vi "liftCellOrPullPatch-v02.vi"(0 "which manipulator":T5(ring), 1 "controls array in":refnum<vi>[](array[refnum]), 5 "LiftCell?":bool, 7 "set pressure (mBar)":dbl format="%#_13g", 11 "error in":errorcluster, 12 "common cluster":T4, 13 "individual controls in":T3, 14 "images":T1) -> (3 "control array out":refnum<vi>[](array[refnum]), 15 "error out":errorcluster)   [LabVIEW 2019]
uses:
  multipatch/controls/multipatch_common_controls_v4.ctl
  machine_vision/controls/transform_cluster_actuator.ctl
  machine_vision/coordinate model vis/transform_properties_actuators.ctl
  pipette cleaning/pressure box/cleaning_soft/controls/actuator_cluster.ctl
  pipette cleaning/pressure box/cleaning_soft/controls/actuator_type.ctl
  pipette cleaning/pressure box/cleaning_soft/controls/pressure_box_control.ctl
  pipette cleaning/pressure box/cleaning_soft/controls/pressure_box_type.ctl
  controls/NH_method.ctl
  multipatch/controls/multipatch_individual_controls_v5.ctl
  controls/memtest_def.ctl
  multipatch/controls/images_controls.ctl
  <vilib>/vision/Image Controls.llb/IMAQ Image.ctl
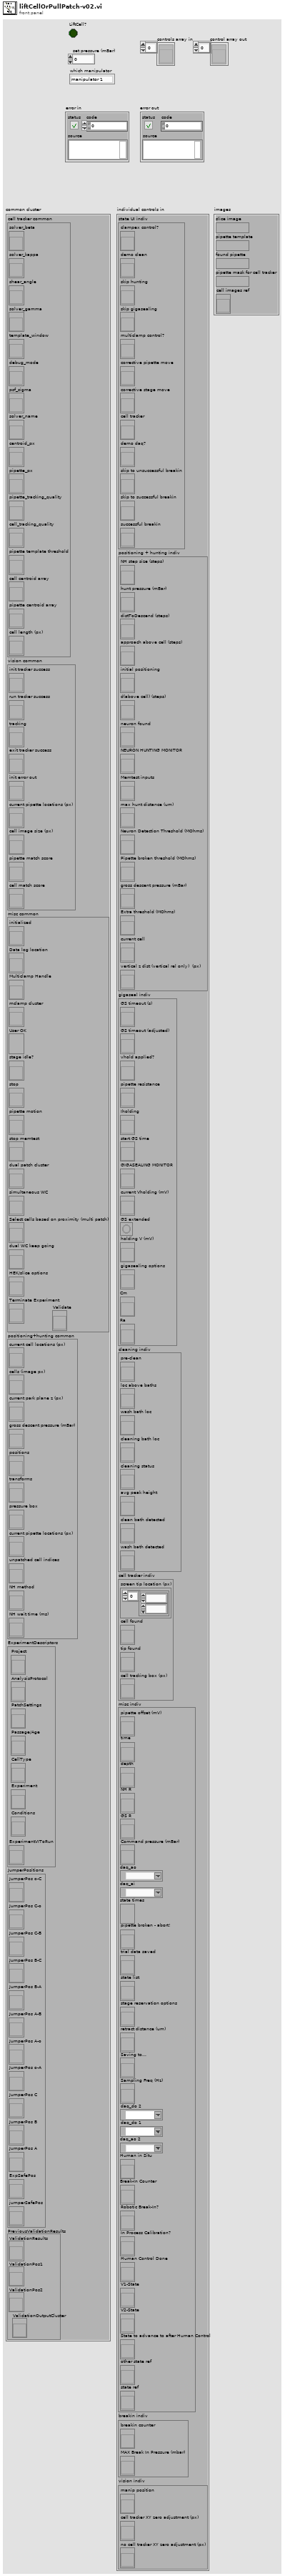
[diagram p1: front panel]
types:
  T1 = typedef "images_controls.ctl" = cluster{"slice image":T2, "pipette template":T2, "found pipette":T2, "pipette mask for cell tracker":T2, "cell images ref":refnum<vi>}
  T2 = typedef "IMAQ Image.ctl" = refnum<image>
  T3 = typedef "multipatch_individual_controls_v5.ctl" = cluster{"state UI indiv":cluster{"clampex control?":refnum<vi>, "demo clean":refnum<vi>, "skip hunting":refnum<vi>, "skip gigasealing":refnum<vi>, "multiclamp control?":refnum<vi>, "corrective pipette move":refnum<vi>, "corrective stage move":refnum<vi>, "cell tracker":refnum<vi>, "demo daq?":refnum<vi>, "skip to unsuccessful breakin":refnum<vi>, "skip to successful breakin":refnum<vi>, "successful breakin":refnum<vi>}, "positioning + hunting indiv":cluster{"NH step size (steps)":refnum<vi>, "hunt pressure (mBar)":refnum<vi>, "distToDescend (steps)":refnum<vi>, "approach above cell (steps)":refnum<vi>, "initial positioning":refnum<vi>, "d(above cell) (steps)":refnum<vi>, "neuron found":refnum<vi>, "NEURON HUNTING MONITOR":refnum<vi>, "Memtest inputs":refnum<vi>, "max hunt distance (um)":refnum<vi>, "Neuron Detection Threshold (MOhms)":refnum<vi>, "Pipette broken threshold (MOhms)":refnum<vi>, "gross descent pressure (mBar)":refnum<vi>, "Extra threshold (MOhms)":refnum<vi>, "current cell":refnum<vi>, "vertical z dist (vertical rel only)  (px)":refnum<vi>}, "gigaseal indiv":cluster{"GS timeout (s)":refnum<vi>, "GS timeout (adjusted)":refnum<vi>, "vhold applied?":refnum<vi>, "pipette resistance":refnum<vi>, "Iholding":refnum<vi>, "start GS time":refnum<vi>, "GIGASEALING MONITOR":refnum<vi>, "current Vholding (mV)":refnum<vi>, "GS extended":refnum<vi>, "holding V (mV)":refnum<vi>, "gigasealing options":refnum<vi>, "Cm":refnum<vi>, "Ra ":refnum<vi>}, "cleaning indiv":cluster{"pre-clean":refnum<vi>, "loc above baths":refnum<vi>, "wash bath loc":refnum<vi>, "cleaning bath loc":refnum<vi>, "cleaning status":refnum<vi>, "avg peak height":refnum<vi>, "clean bath detected":refnum<vi>, "wash bath detected":refnum<vi>}, "cell tracker indiv":cluster{"screen tip location (px)":refnum<vi>, "cell found":refnum<vi>, "tip found":refnum<vi>, "cell tracking box (px)":refnum<vi>}, "misc indiv":cluster{"pipette offset (mV)":refnum<vi>, "time":refnum<vi>, "depth":refnum<vi>, "NH R":refnum<vi>, "GS R":refnum<vi>, "Command pressure (mBar)":refnum<vi>, "daq_ao":tag, "daq_ai":tag, "state times":refnum<vi>, "pipette broken - abort!":refnum<vi>, "trial data saved":refnum<vi>, "state list":refnum<vi>, "stage reservation options":refnum<vi>, "retract distance (um)":refnum<vi>, "Saving to...":refnum<vi>, "Sampling Freq (Hz)":refnum<vi>, "daq_do 2":tag, "daq_do 1":tag, "daq_ao 2":tag, "Human in Situ":refnum<vi>, "Break-In Counter":refnum<vi>, "Robotic Break-In?":refnum<vi>, "In Process Calibration?":refnum<vi>, "Human Control Done":refnum<vi>, "V1-State":refnum<vi>, "V2-State":refnum<vi>, "State to advance to after Human Control":refnum<vi>, "other state ref":refnum<vi>, "state ref":refnum<vi>}, "breakin indiv":cluster{"breakin counter":refnum<vi>, "MAX Break In Pressure (mbar)":refnum<vi>}, "vision indiv":cluster{"manip position":refnum<vi>, "cell tracker XY zero adjustment (px)":refnum<vi>, "no cell tracker XY zero adjustment (px)":refnum<vi>}}
  T4 = typedef "multipatch_common_controls_v4.ctl" = cluster{"cell tracker common":cluster{"solver_beta":refnum<vi>, "solver_kappa":refnum<vi>, "shear_angle":refnum<vi>, "solver_gamma":refnum<vi>, "template_window":refnum<vi>, "debug_mode":refnum<vi>, "psf_sigma":refnum<vi>, "solver_name":refnum<vi>, "centroid_px":refnum<vi>, "pipette_px":refnum<vi>, "pipette_tracking_quality":refnum<vi>, "cell_tracking_quality":refnum<vi>, "pipette template threshold":refnum<vi>, "cell centroid array":refnum<vi>, "pipette centroid array":refnum<vi>, "cell length (px)":refnum<vi>}, "vision common":cluster{"init tracker success":refnum<vi>, "run tracker success":refnum<vi>, "tracking":refnum<vi>, "exit tracker success":refnum<vi>, "init error out":refnum<vi>, "current pipette locations (px)":refnum<vi>, "cell image size (px)":refnum<vi>, "pipette match score":refnum<vi>, "cell match score":refnum<vi>}, "misc common":cluster{"initialized":refnum<vi>, "Data log location":refnum<vi>, "Multiclamp Handle":refnum<vi>, "mclamp cluster":refnum<vi>, "User OK":refnum<vi>, "stage idle?":refnum<vi>, "stop":refnum<vi>, "pipette motion":refnum<vi>, "stop memtest":refnum<vi>, "dual patch cluster":refnum<vi>, "simultaneous WC":refnum<vi>, "Select cells based on proximity (multi patch)":refnum<vi>, "dual WC keep going":refnum<vi>, "HEK/slice options":refnum<vi>, "Terminate Experiment":refnum<vi>, "Validate":refnum<vi>}, "positioning+hunting common":cluster{"current cell locations (px)":refnum<vi>, "cells (image px)":refnum<vi>, "current park plane z (px)":refnum<vi>, "gross descent pressure (mBar)":refnum<vi>, "positions":refnum<vi>, "transforms":refnum<vi>, "pressure box":refnum<vi>, "current pipette locations (px)":refnum<vi>, "unpatched cell indices":refnum<vi>, "NH method":refnum<vi>, "NH wait time (ms)":refnum<vi>}, "ExperimentDescriptors":cluster{"Project":refnum<vi>, "AnalysisProtocol":refnum<vi>, "PatchSettings":refnum<vi>, "Passage/Age":refnum<vi>, "CellType":refnum<vi>, "Experiment":refnum<vi>, "Conditions":refnum<vi>, "ExperimentVIToRun":refnum<vi>}, "JumperPositions":cluster{"JumperPos o-C":refnum<vi>, "JumperPos C-o":refnum<vi>, "JumperPos C-B":refnum<vi>, "JumperPos B-C":refnum<vi>, "JumperPos B-A":refnum<vi>, "JumperPos A-B":refnum<vi>, "JumperPos A-o":refnum<vi>, "JumperPos o-A":refnum<vi>, "JumperPos C":refnum<vi>, "JumperPos B":refnum<vi>, "JumperPos A":refnum<vi>, "ExpSafePos":refnum<vi>, "jumperSafePos":refnum<vi>}, "PreviousValidationResults":cluster{"ValidationResults":refnum<vi>, "ValidationPos1":refnum<vi>, "ValidationPos2":refnum<vi>, "ValidationOutputCluster":refnum<vi>}}
  T5 = enum16{"manipulator 1", "manipulator 2", "manipulator 3", "manipulator 4"}
  T6 = cluster{"current stage pos (steps)":refnum<vi>, "current manip 1 pos (steps)":refnum<vi>, "current manip 2 pos (steps)":refnum<vi>, "current manip 3 pos (steps)":refnum<vi>, "current manip 4 pos (steps)":refnum<vi>}
  T7 = typedef "pressure_box_control.ctl" = cluster{"Pressure box COM":refnum<visa-resource-name>, "pressure box type":T8, "High pos pressure (mBar)":dbl, "Low pos pressure (mBar)":dbl, "Vacuum pressure (mBar)":dbl, "calibration":enum16{"PA_vacPump", "PA_venturi", "Neuromatics", "ilyaRig", "mightenRig"}}
  T8 = typedef "pressure_box_type.ctl" = enum16{"Neuromatics", "ProportionAir", "Demo box", "N-ProportionAir"}
  T9 = typedef "transform_cluster_actuator.ctl" = cluster{"s":refnum<vi>, "manip 1":refnum<vi>, "manip 2":refnum<vi>, "manip 3":refnum<vi>, "manip 4":refnum<vi>}
  T10 = typedef "scope_motion.ctl" = enum16{"superSlow", "fast", "slow", "find slice speed", "slow_dualPatch"}
  T11 = typedef "transform_properties_actuators.ctl" = cluster{"theta (deg)":dbl, "X sc factor (px/step)":dbl, "Y sc factor (px/step)":dbl, "zero loc (x,y,z)":dbl[], "flip y?":bool, "flip x?":bool, "gamma (deg)":dbl, "flip z?":bool, "Z sc factor (px/step)":dbl, "actuator":T12, "safe space (steps)":i32[]}
  T12 = typedef "actuator_cluster.ctl" = cluster{"Actuator COM":refnum<visa-resource-name>, "Actuator type":T13}
  T13 = typedef "actuator_type.ctl" = enum16{"Scientifica", "Sutter", "Demo", "Off"}
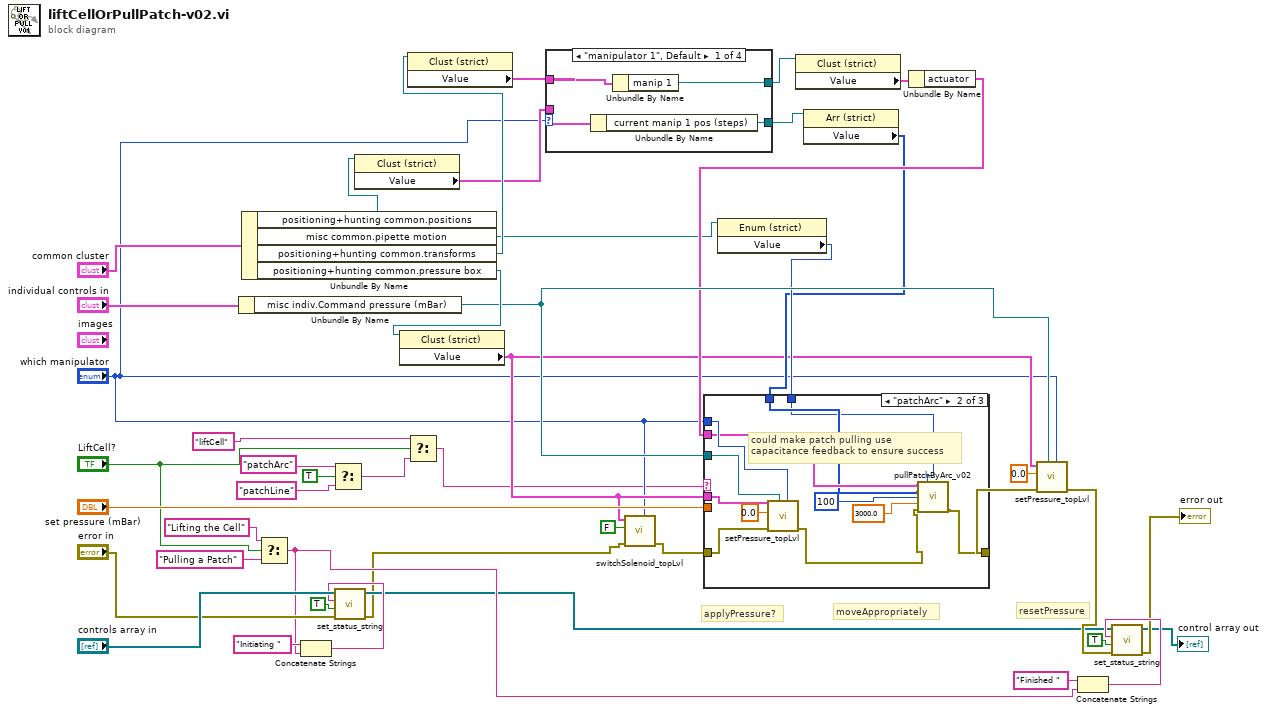
[diagram p0: block diagram]
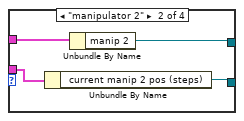
[diagram p2: hidden frame]
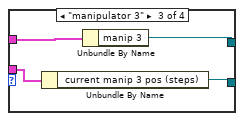
[diagram p3: hidden frame]
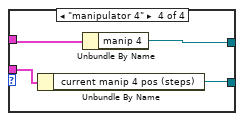
[diagram p4: hidden frame]
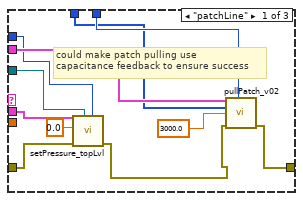
[diagram p5: hidden frame]
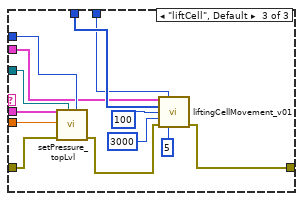
[diagram p6: hidden frame]
diagram:
  # "resetPressure"
  # "moveAppropriately"
  # "applyPressure?"
  n1 = Unbundle By Name("individual controls in") -> ("misc indiv.Command pressure (mBar)"=w40:refnum<vi>)
  n2 = Unbundle By Name("common cluster") -> ("positioning+hunting common.positions"=w31:refnum<vi>, "misc common.pipette motion"=w33:refnum<vi>, "positioning+hunting common.transforms"=w34:refnum<vi>, "positioning+hunting common.pressure box"=w42:refnum<vi>)
  n3 = Select(t="Lifting the Cell" ("status string in"), s="LiftCell?", f="Pulling a Patch") -> (s? t:f=w15:string)
  n4 = Concatenate Strings("Initiating " ("string"), w15) -> (w22:string)
  n5 = Select(t="patchArc" ("status string in"), s=TRUE, f="patchLine" ("status string in")) -> (s? t:f=w5:string)
  n6 = call "set_status_string.vi"("error in"="error in", "new line?"=TRUE, "status string in"=w22, "controls array"="controls array in") -> ("error out"=w11:errorcluster, "controls array out"=w14:refnum<vi>[])  [unwired: 6 in]
  n7 = property class="Clust (strict)"(reference=w31) -> ("Value"=w30:T6)  [unwired: 1 in, 2 out]
  n8 = property class="Clust (strict)"(reference=w42) -> ("Value"=w10:T7)  [unwired: 1 in, 2 out]
  n9 = property class="Clust (strict)"(reference=w34) -> ("Value"=w38:T9)  [unwired: 1 in, 2 out]
  n10 = Select(t="liftCell" ("status string in"), s="LiftCell?", f=w5) -> (s? t:f=w1:string)
  n11 = case shown="\"manipulator 1\", Default" "which manipulator" {
    tunnel: w38 -> [w49 w53 w57 w61]
    tunnel: [w48 w52 w56 w60] -> w37
    tunnel: w30 -> [w47 w51 w55 w59]
    tunnel: [w46 w50 w54 w58] -> w29
    frame "manipulator 1", Default {
      n12 = Unbundle By Name(w47) -> ("current manip 1 pos (steps)"=w46:refnum<vi>)
      n13 = Unbundle By Name(w49) -> ("manip 1"=w48:refnum<vi>)
    }
    frame "manipulator 2" {
      n14 = Unbundle By Name(w51) -> ("current manip 2 pos (steps)"=w50:refnum<vi>)
      n15 = Unbundle By Name(w53) -> ("manip 2"=w52:refnum<vi>)
    }
    frame "manipulator 3" {
      n16 = Unbundle By Name(w55) -> ("current manip 3 pos (steps)"=w54:refnum<vi>)
      n17 = Unbundle By Name(w57) -> ("manip 3"=w56:refnum<vi>)
    }
    frame "manipulator 4" {
      n18 = Unbundle By Name(w59) -> ("current manip 4 pos (steps)"=w58:refnum<vi>)
      n19 = Unbundle By Name(w61) -> ("manip 4"=w60:refnum<vi>)
    }
  }
  n20 = call "switchSolenoid_topLvl.vi"("which manipulator"="which manipulator", "error in (no error)"=w11, "solenoidSwitch (T:atm; F: Reg)"=FALSE, "Pressure box control in"=w10) -> ("error out"=w8:errorcluster)  [unwired: 6 in, 1 out]
  n21 = property class="Enum (strict)"(reference=w33) -> ("Value"=w32:T10)  [unwired: 1 in, 2 out]
  n22 = property class="Clust (strict)"(reference=w37) -> ("Value"=w36:T11)  [unwired: 1 in, 2 out]
  n23 = property class="Arr (strict)"(reference=w29) -> ("Value"=w28:i32[])  [unwired: 1 in, 2 out]
  n24 = Unbundle By Name(w36) -> ("actuator"=w35:T12)
  n25 = case shown="\"patchArc\"" w1 {
    tunnel: w8 -> [w67 w84 w93]
    tunnel: [w70 w75 w90] -> w41
    tunnel: "set pressure (mBar)" -> [_ _ w97]
    tunnel: "which manipulator" -> [w63 w81 w96]
    tunnel: w40 -> [w64 w82 w95]
    tunnel: w10 -> [w65 w83 w94]
    tunnel: w35 -> [w72 w80 w88]
    tunnel: w32 -> [w69 w76 w89]
    tunnel: w28 -> [w68 w79 w92]
    frame "patchLine" {
      # "could make patch pulling use \ncapacitance feedback to ensure success"
      n26 = call "setPressure_topLvl.vi"("which manipulator"=w63, "Slide Refnum"=w64, "error in"=w67, "set pressure (mBar)"=0.0, "Pressure box control in"=w65) -> ("error out"=w66:errorcluster)  [unwired: 5 in, 1 out]
      n27 = call "pullPatch_v02.vi"("manp in"=w72, "reset motion"=w69, "Current Position"=w68, "retract distance (um)"=3000.0, "error in"=w66) -> ("error out"=w70:errorcluster)  [unwired: 9 in, 1 out]
    }
    frame "patchArc" {
      # "could make patch pulling use \ncapacitance feedback to ensure success"
      n28 = call "setPressure_topLvl.vi"("which manipulator"=w81, "Slide Refnum"=w82, "error in"=w84, "set pressure (mBar)"=0.0, "Pressure box control in"=w83) -> ("error out"=w77:errorcluster)  [unwired: 5 in, 1 out]
      n29 = call "pullPatchByArc_v02.vi"("manp in"=w80, "reset motion"=w76, "Current Position"=w79, "Steps"=100, "Final Distance (steps)"=3000.0 ("retract distance (um)"), "error in"=w77) -> ("error out"=w75:errorcluster)  [unwired: 8 in, 1 out]
    }
    frame "liftCell", Default {
      n30 = call "setPressure_topLvl.vi"("which manipulator"=w96, "Slide Refnum"=w95, "error in"=w93, "set pressure (mBar)"=w97, "Pressure box control in"=w94) -> ("error out"=w91:errorcluster)  [unwired: 5 in, 1 out]
      n31 = call "liftingCellMovement_v01.vi"("manp in"=w88, "reset motion"=w89, "Current Position"=w92, "NumberOfIncrements"=100 ("NumberOfSteps"), "Final Distance (steps)"=3000 ("Final Distance"), "error in"=w91, "NumberOfSpirals"=5) -> ("error out"=w90:errorcluster)  [unwired: 7 in, 1 out]
    }
  }
  n32 = call "setPressure_topLvl.vi"("which manipulator"="which manipulator", "Slide Refnum"=w40, "error in"=w41, "set pressure (mBar)"=0.0, "Pressure box control in"=w10) -> ("error out"=w17:errorcluster)  [unwired: 5 in, 1 out]
  n33 = Concatenate Strings("Finished " ("string"), w15) -> (w19:string)
  n34 = call "set_status_string.vi"("error in"=w17, "new line?"=TRUE, "status string in"=w19, "controls array"=w14) -> ("error out"=→"error out":errorcluster, "controls array out"=→"control array out":refnum<vi>[])  [unwired: 6 in]
